vi "StringHashFunction.vi"(11 "Key":string) -> (3 "Hash":i32)   [LabVIEW 2017]
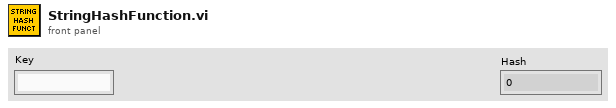
[diagram p1: front panel]
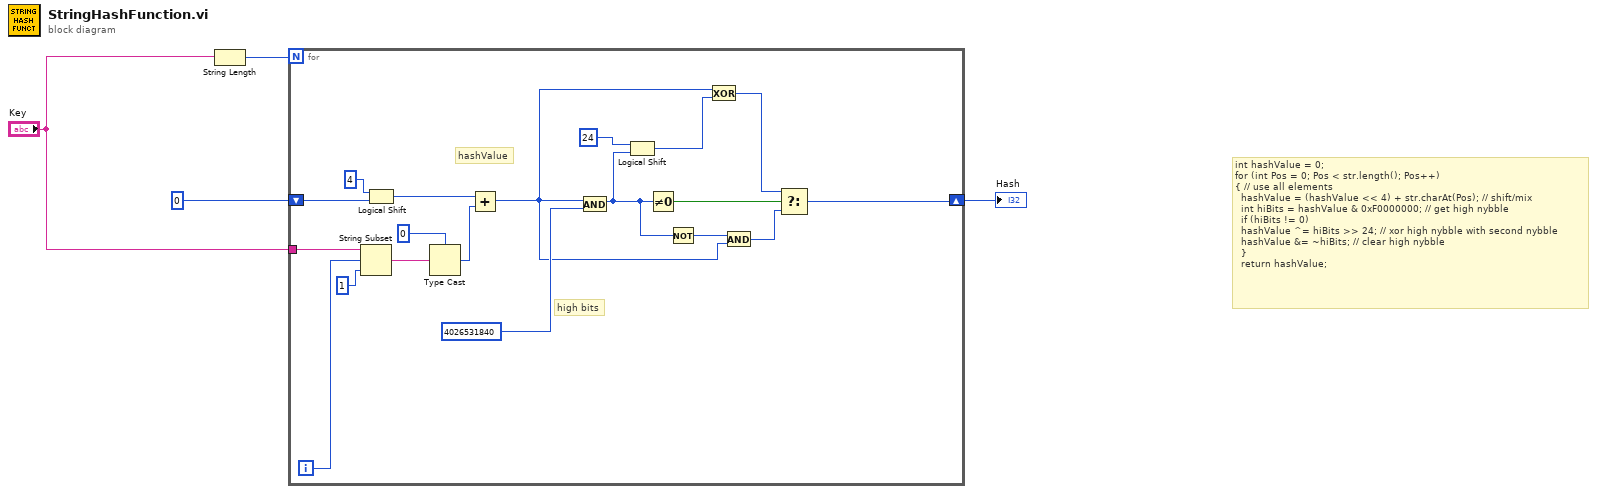
[diagram p0: block diagram]
diagram:
  # "int hashValue = 0;\nfor (int Pos = 0; Pos < str.length(); Pos++) \n{ // use all elements\n\t\thashValue = (hashValue << 4) + str.charAt(Pos); // shift/mix\n\t\tint hiBits = hashValue & 0xF0000000; // get high nybble\n\t\tif (hiBits != 0)\n\t\thashValue ^= hiBits >> 24; // xor high nybble with second nybble\n\t\thashValue &= ~hiBits; // clear high nybble\n\t\t}\n\t\treturn hashValue;"
  n1 = String Length(string="Key") -> (length=w4:i32)
  n2 = for {
    N: w4 -> [_]
    tunnel: "Key" -> [w20]
    shift-right: [w5] -> w1
    shift-left: 0 -> [w23]
    i -> [w19]
    # "hashValue"
    # "high bits"
    n3 = String Subset(string=w20, offset (0)=w19, length (rest)=1 ("length (rest)")) -> (substring=w17:string)
    n4 = Logical Shift(y=i16 4, x=w23) -> (x << y=w21:u32)
    n5 = Type Cast(type=0, x=w17) -> (*(type *) &x=w15:i32)
    n6 = Add(x=w21, y=w15) -> (x+y=w7:u32)
    n7 = And(x=w7, y=u32 4026531840) -> (x .and. y?=w9:u32)
    n8 = Logical Shift(y=i16 24, x=w9) -> (x << y=w11:u32)
    n9 = Not Equal To 0?(x=w9) -> (x != 0?=w13:bool)
    n10 = Not(x=w9) -> (.not. x?=w8:u32)
    n11 = Exclusive Or(1:w11, 2:w7) -> (0:w10:u32)
    n12 = And(x=w8, y=w7) -> (x .and. y?=w6:u32)
    n13 = Select(t=w10, s=w13, f=w6) -> (s? t:f=w5:u32)
  }
  "Hash" <- w1
